vi "字符串操作函数（三）.vi"() -> ()   [LabVIEW 2010]
panel:
  out "格式化输出字符串":string
  out "系统日期时间":string
  out "替换结果":string
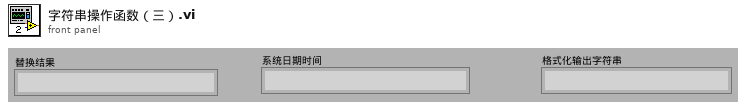
[diagram p1: front panel]
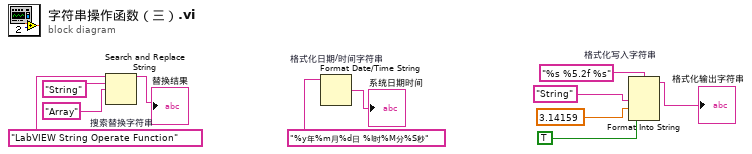
[diagram p0: block diagram]
diagram:
  n1 = Search and Replace String "搜索替换字符串"(input string="LabVIEW String Operate Function", search string="String", replace string="Array") -> (result string=→"替换结果":string)  [unwired: 5 in, 3 out]
  n2 = Format Date/Time String "格式化日期/时间字符串"(time format string (%c)="%y年%m月%d日 %I时%M分%S秒") -> (date/time string=→"系统日期时间":string)  [unwired: 2 in]
  n3 = Format Into String "格式化写入字符串"(format string="%s %5.2f %s", "String", 3.14159, TRUE) -> (resulting string=→"格式化输出字符串":string)  [unwired: 2 in, 1 out]
